vi "AutoAlign_P612_Jan5th2014.vi"() -> ()   [LabVIEW 2014]
uses:
  Controls/StageStates.ctl
panel:
  in  "Align":bool
  in  "Exit":bool
  out "Image":sgl[][](graph)
  out "Aligned":bool
  in  "Repeat":bool
  in  "Quit":bool
  out "Sample":cluster{"X":dbl, "Y":dbl}[](graph)
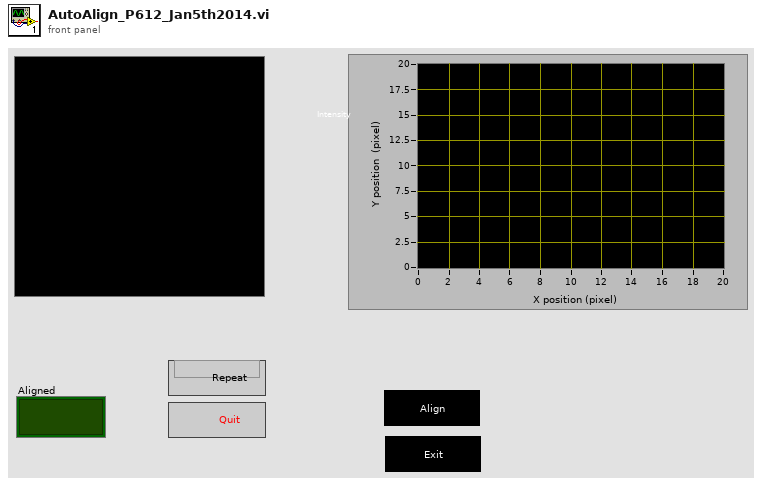
[diagram p1: front panel]
types:
  T1 = typedef "StageStates.ctl" = enum16{"POSITION", "MVR", "MOVE", "HALT", "ONTARGET", "ERROR", "EXIT", "HOME", "ZEROPOS", "NANOPOS", "QUIT", "ANALOG"}
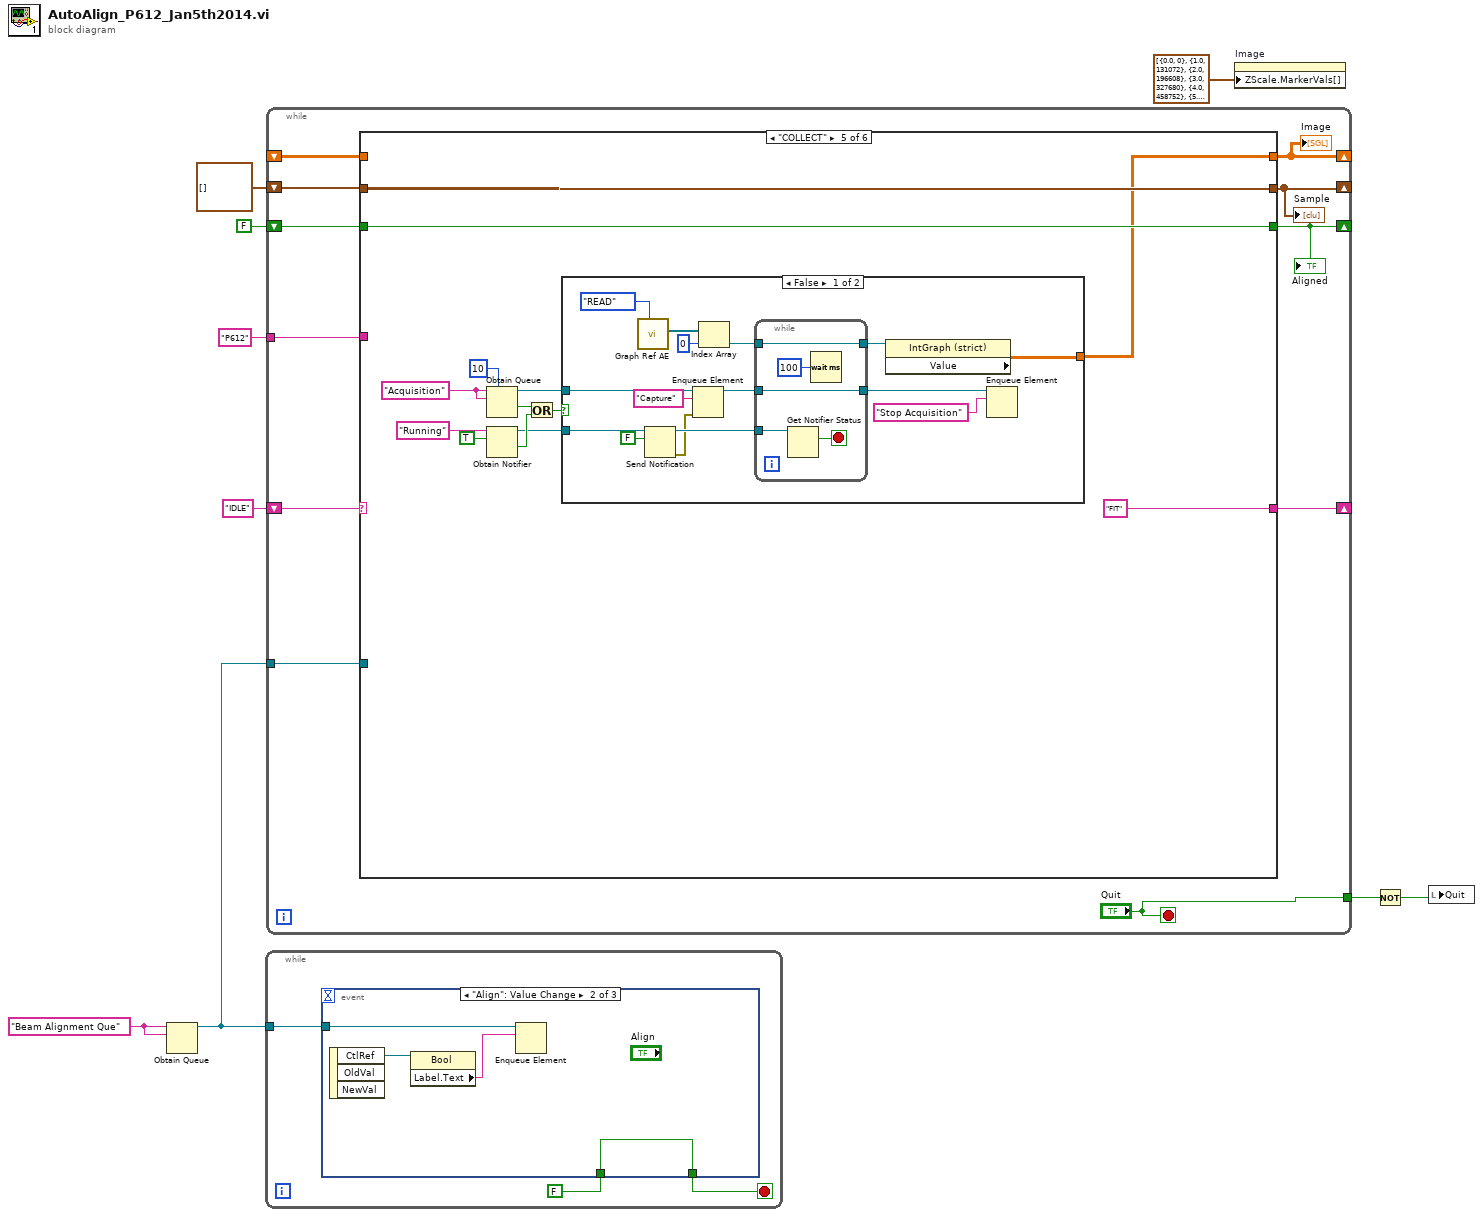
[diagram p0: block diagram]
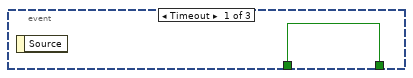
[diagram p2: hidden frame]
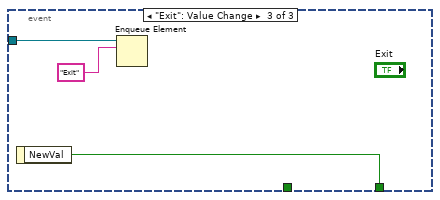
[diagram p3: hidden frame]
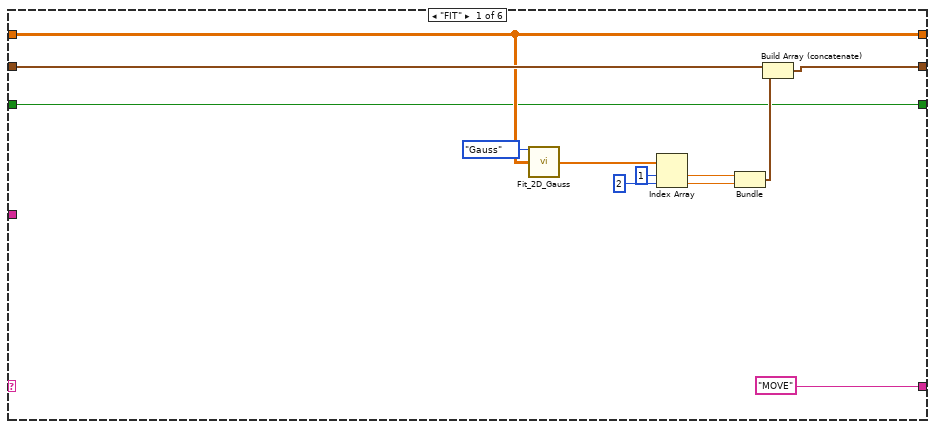
[diagram p4: hidden frame]
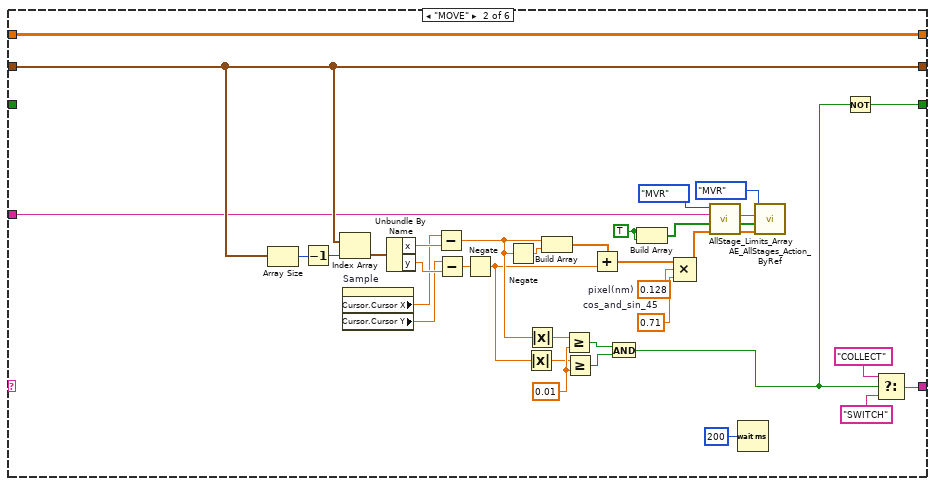
[diagram p5: hidden frame]
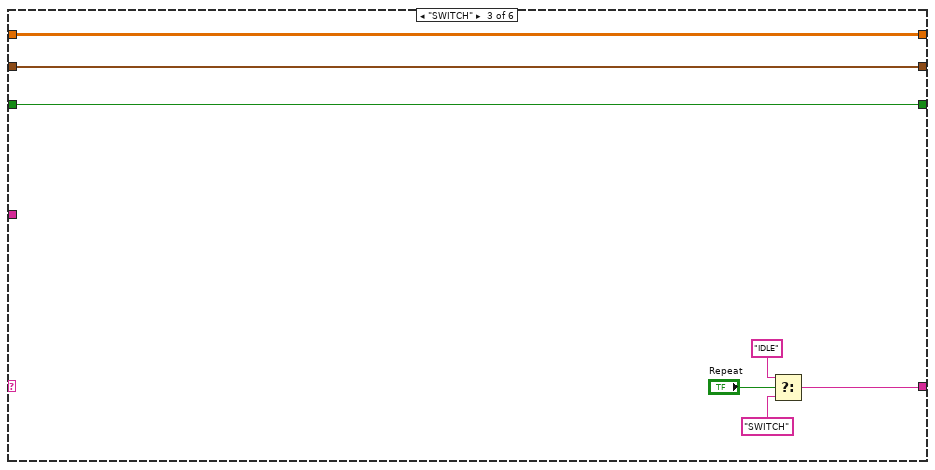
[diagram p6: hidden frame]
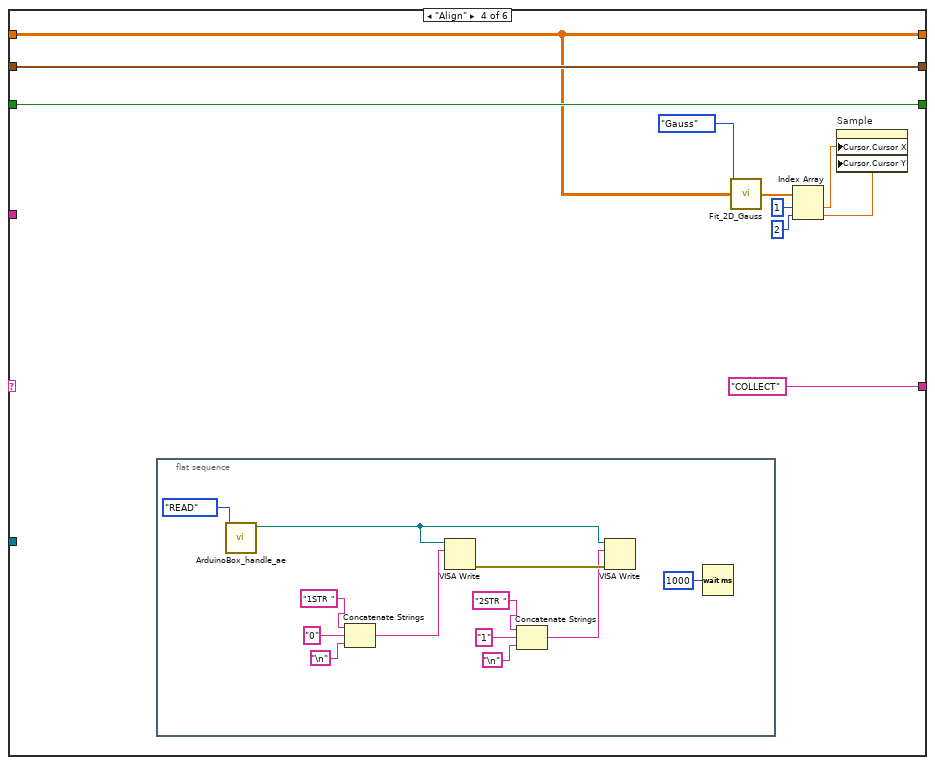
[diagram p7: hidden frame]
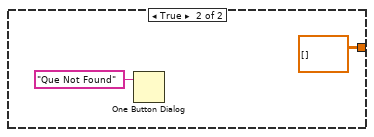
[diagram p8: hidden frame]
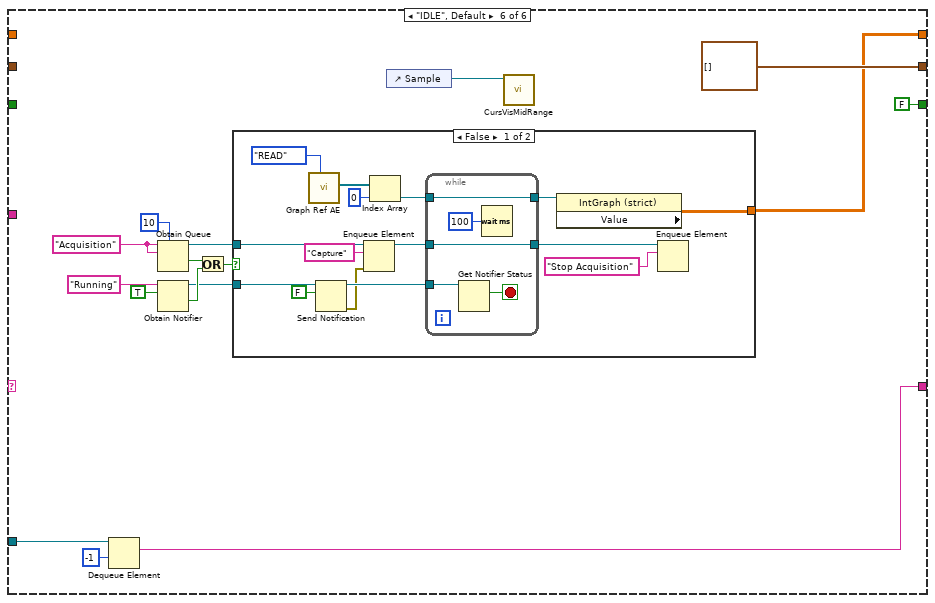
[diagram p9: hidden frame]
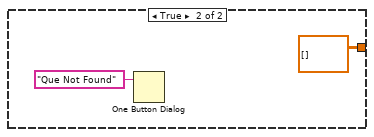
[diagram p10: hidden frame]
diagram:
  w2 = "Beam Alignment Que" ("name (unnamed)")
  n1 = Obtain Queue(name (unnamed)=w2, element data type=w2) -> (queue out=w1:refnum<queue>)  [unwired: 3 in, 2 out]
  n2 = while {
    tunnel: w1 -> [w12]
    stop <- w10 stop-if-true
    n3 = event shown="[1] \"Align\": Value Change" {
      selector: _ -> [_ _ _]
      dyn-events: _ -> [_ _ _]
      timeout: _ -> [_ _ _]
      tunnel: w12 -> [_ w15 w20]
      tunnel: FALSE -> [w13 w14 _]
      tunnel: [w13 w14 w18] -> w10
      event Timeout {
        n4 = event-data() -> ()  [unwired: 1 in, 1 out]
      }
      event "Align": Value Change {
        n5 = event-data() -> ("CtlRef"=w17:refnum<vi>)  [unwired: 1 in, 2 out]
        n6 = property class="Bool"(reference=w17) -> ("Label.Text"=w16:string)  [unwired: 1 in, 2 out]
        n7 = Enqueue Element(queue=w15, element=w16) -> ()  [unwired: 2 in, 3 out]
      }
      event "Exit": Value Change {
        n8 = event-data() -> ("NewVal"=w18:bool)  [unwired: 1 in]
        n9 = Enqueue Element(queue=w20, element="Exit") -> ()  [unwired: 2 in, 3 out]
      }
    }
  }
  n10 = while {
    shift-right: [w22] -> _
    shift-left: _ -> [w31]
    shift-right: [w30] -> _
    shift-left: cluster{"x":dbl, "y":dbl}[] [] ("XY chart data") -> [w24]
    shift-right: [w29] -> _
    shift-left: "IDLE" -> [w26]
    shift-right: [w27] -> _
    shift-left: FALSE -> [w28]
    tunnel: "P612" ("StageID") -> [w25]
    tunnel: ["Quit"] -> w5
    tunnel: w1 -> [w21]
    stop <- "Quit" stop-if-true
    n11 = case shown="\"COLLECT\"" w26 {
      tunnel: [w39 w80 w85 w88 w110 w145] -> w22
      tunnel: w31 -> [w39 w80 w85 w88 _ _]
      tunnel: w24 -> [w41 w54 w86 w95 w122 _]
      tunnel: [w40 w54 w86 w95 w122 cluster{"x":dbl, "y":dbl}[] [] ("XY chart data")] -> w30
      tunnel: w25 -> [_ w47 _ _ _ _]
      tunnel: ["MOVE" w67 w82 "COLLECT" "FIT" w155] -> w29
      tunnel: w28 -> [w37 _ w87 w97 w121 _]
      tunnel: [w37 w52 w87 w97 w121 FALSE] -> w27
      tunnel: w21 -> [_ _ _ _ _ w157]
      frame "FIT" {
        n12 = call "Fit_2D_Gauss.vi"("Enum"=enum16{"Gauss", "Lorentz"}."Gauss", "Image IN"=w39) -> ("Fit Parameters"=w43:dbl[])  [unwired: 12 in, 1 out]
        n13 = Index Array(array=w43, index #1=1 ("index"), index #2=2 ("index")) -> (element #1=w34:dbl, element #2=w33:dbl)
        n14 = Bundle("Numeric"=w34, "Numeric"=w33) -> (w42:cluster{"Numeric":dbl, "Numeric":dbl})  [unwired: 1 in]
        n15 = Build Array (concatenate)(w41, w42) -> (w40:cluster{"Numeric":dbl, "Numeric":dbl}[])
      }
      frame "MOVE" {
        w66 = 0.71  # cos_and_sin_45
        w79 = 0.01 ("y")
        w78 = 0.128  # pixel(nm)
        w77 = TRUE
        n16 = Array Size(array=w54) -> (size(s)=w72:i32)
        n17 = Decrement(x=w72) -> (x-1=w65:i32)
        n18 = Index Array(array=w54, index=w65) -> (element=w73:cluster{"x":dbl, "y":dbl})
        n19 = property on="Sample" class="XYGraph (strict)"() -> ("Cursor.Cursor X"=w71:dbl, "Cursor.Cursor Y"=w70:dbl)  [unwired: 2 in, 2 out]
        n20 = Unbundle By Name(w73) -> ("x"=w74:dbl, "y"=w75:dbl)
        n21 = Subtract(x=w71, y=w74) -> (x-y=w61:dbl)
        n22 = Subtract(x=w70, y=w75) -> (x-y=w62:dbl)
        n23 = Negate(x=w62) -> (-x=w58:dbl)
        n24 = Negate(x=w61) -> (-x=w60:dbl)
        n25 = Absolute Value(x=w58) -> (abs(x)=w63:dbl)
        n26 = Absolute Value(x=w61) -> (abs(x)=w64:dbl)
        n27 = Build Array(w61, w60) -> (w59:dbl[])
        n28 = Greater Or Equal?(x=w64, y=w79) -> (x >= y?=w56:bool)
        n29 = Greater Or Equal?(x=w63, y=w79) -> (x >= y?=w55:bool)
        n30 = Add(x=w59, y=w58) -> (x+y=w57:dbl[])
        n31 = And(x=w56, y=w55) -> (x .and. y?=w53:bool)
        n32 = Build Array(w77, w77) -> (w46:bool[])
        n33 = Compound Arithmetic op=MULTIPLY(w57, w78, w66) -> (w48:dbl[])
        n34 = call "AllStage_Limits_Array.vi"("Step(um)/Position(units)"=w48, "Axis"=w46, "Stage ID"=w47, "MOVE/MVR"=enum16{"MOVE", "MVR"}."MVR") -> ("Positions"=w49:dbl[], "Boolean Array"=w50:bool[], "Stage ID"=w51:string)  [unwired: 5 in]
        n35 = Wait (ms)(milliseconds to wait=u32 200) -> ()  [unwired: 1 out]
        n36 = call "AE_AllStages_Action_ByRef.vi"("Positions"=w49, "Axis"=w50, "Stage ID"=w51, "Action"=StageStates."MVR") -> ()  [unwired: 4 in, 4 out]
        n37 = Not(x=w53) -> (.not. x?=w52:bool)
        n38 = Select(t="COLLECT", s=w53, f="SWITCH") -> (s? t:f=w67:string)
      }
      frame "SWITCH" {
        n39 = Select(t="IDLE", s="Repeat", f="SWITCH") -> (s? t:f=w82:string)
      }
      frame "Align" {
        n40 = flat-sequence {
          frame #0 {
            n41 = call "ArduinoBox_handle_ae.vi"("Enum"=enum16{"WRITE", "READ"}."READ") -> ("VISA resource Out"=w103:refnum<visa-resource-name>)  [unwired: 10 in]
            n42 = Concatenate Strings("1STR ", "0" ("string"), "\n") -> (w106:string)
            n43 = VISA Write(VISA resource name=w103, write buffer=w106) -> (error out=w104:errorcluster)  [unwired: 1 in, 2 out]
            n44 = Concatenate Strings("2STR ", "1" ("string"), "\n") -> (w99:string)
            n45 = VISA Write(VISA resource name=w103, write buffer=w99, error in (no error)=w104) -> ()  [unwired: 3 out]
            n46 = Wait (ms)(milliseconds to wait=u32 1000) -> ()  [unwired: 1 out]
          }
        }
        n47 = call "Fit_2D_Gauss.vi"("Enum"=enum16{"Gauss", "Lorentz"}."Gauss", "Image IN"=w88) -> ("Fit Parameters"=w94:dbl[])  [unwired: 12 in, 1 out]
        n48 = Index Array(array=w94, index #1=1 ("index"), index #2=2 ("index")) -> (element #1=w91:dbl, element #2=w90:dbl)
        n49 = property on="Sample" class="XYGraph (strict)"("Cursor.Cursor X"=w91, "Cursor.Cursor Y"=w90) -> ()  [unwired: 2 in, 2 out]
      }
      frame "COLLECT" {
        w114 = "Acquisition" ("name (unnamed)")
        n50 = Obtain Queue(max queue size (-1, unlimited)=10, name (unnamed)=w114, element data type=w114) -> (queue out=w111:refnum<queue>, created new?=w117:bool)  [unwired: 2 in, 1 out]
        n51 = Obtain Notifier(name (unnamed)="Running", notification data type=TRUE) -> (notifier out=w112:refnum<notifier>, created new?=w118:bool)  [unwired: 2 in, 1 out]
        n52 = Or(x=w117, y=w118) -> (x .or. y?=w119:bool)
        n53 = case shown="False" w119 {
          tunnel: w111 -> [w126 _]
          tunnel: w112 -> [w124 _]
          tunnel: [w123 sgl[][] [] ("Value")] -> w110
          frame False {
            n54 = call "Graph Ref AE.vi"("Action"=enum16{"READ", "WRITE"}."READ") -> ("Graph Ref Out"=w134:refnum<vi>[])  [unwired: 10 in]
            n55 = Send Notification(notification=FALSE, notifier=w124) -> (notifier out=w129:refnum<notifier>, error out=w128:errorcluster)  [unwired: 1 in]
            n56 = Enqueue Element(queue=w126, element="Capture", error in (no error)=w128) -> (queue out=w130:refnum<queue>)  [unwired: 1 in, 2 out]
            n57 = Index Array(array=w134, index=0) -> (element=w136:refnum<vi>)
            n58 = while {
              tunnel: w129 -> [w142]
              tunnel: [w140] -> w131
              tunnel: w130 -> [w140]
              tunnel: [w139] -> w137
              tunnel: w136 -> [w139]
              stop <- w141 stop-if-true
              n59 = Get Notifier Status(notifier=w142) -> (current notification=w141:bool)  [unwired: 1 in, 4 out]
              n60 = Wait (ms)(milliseconds to wait=u32 100) -> ()  [unwired: 1 out]
            }
            n61 = property class="IntGraph (strict)"(reference=w137) -> ("Value"=w123:sgl[][])  [unwired: 1 in, 2 out]
            n62 = Enqueue Element(queue=w131, element="Stop Acquisition" ("f")) -> ()  [unwired: 2 in, 3 out]
          }
          frame True {
            n63 = One Button Dialog(message="Que Not Found") -> ()  [unwired: 1 in, 1 out]
          }
        }
      }
      frame "IDLE", Default {
        w149 = "Acquisition" ("name (unnamed)")
        n64 = Dequeue Element(queue=w157, timeout in ms (-1)=-1) -> (element=w155:string)  [unwired: 1 in, 3 out]
        n65 = Obtain Queue(max queue size (-1, unlimited)=10, name (unnamed)=w149, element data type=w149) -> (queue out=w146:refnum<queue>, created new?=w152:bool)  [unwired: 2 in, 1 out]
        n66 = Obtain Notifier(name (unnamed)="Running", notification data type=TRUE) -> (notifier out=w147:refnum<notifier>, created new?=w153:bool)  [unwired: 2 in, 1 out]
        n67 = Or(x=w152, y=w153) -> (x .or. y?=w154:bool)
        n68 = case shown="False" w154 {
          tunnel: w146 -> [w164 _]
          tunnel: w147 -> [w162 _]
          tunnel: [w161 sgl[][] [] ("Value")] -> w145
          frame False {
            n69 = call "Graph Ref AE.vi"("Action"=enum16{"READ", "WRITE"}."READ") -> ("Graph Ref Out"=w172:refnum<vi>[])  [unwired: 10 in]
            n70 = Send Notification(notification=FALSE, notifier=w162) -> (notifier out=w167:refnum<notifier>, error out=w166:errorcluster)  [unwired: 1 in]
            n71 = Enqueue Element(queue=w164, element="Capture", error in (no error)=w166) -> (queue out=w168:refnum<queue>)  [unwired: 1 in, 2 out]
            n72 = Index Array(array=w172, index=0) -> (element=w174:refnum<vi>)
            n73 = while {
              tunnel: w167 -> [w180]
              tunnel: [w178] -> w169
              tunnel: w168 -> [w178]
              tunnel: [w177] -> w175
              tunnel: w174 -> [w177]
              stop <- w179 stop-if-true
              n74 = Get Notifier Status(notifier=w180) -> (current notification=w179:bool)  [unwired: 1 in, 4 out]
              n75 = Wait (ms)(milliseconds to wait=u32 100) -> ()  [unwired: 1 out]
            }
            n76 = property class="IntGraph (strict)"(reference=w175) -> ("Value"=w161:sgl[][])  [unwired: 1 in, 2 out]
            n77 = Enqueue Element(queue=w169, element="Stop Acquisition" ("f")) -> ()  [unwired: 2 in, 3 out]
          }
          frame True {
            n78 = One Button Dialog(message="Que Not Found") -> ()  [unwired: 1 in, 1 out]
          }
        }
        n79 = control-ref of="Sample"() -> (w159:refnum<vi>)
        n80 = call "CursVisMidRange.vi"("XYGraph in"=w159) -> ()  [unwired: 11 in]
      }
    }
    "Sample" <- w30
    "Aligned" <- w27
    "Image" <- w22
  }
  n81 = property on="Image" class="IntGraph (strict)"("ZScale.MarkerVals[]"=cluster{dbl, u32}[] [{0.0, 0}, {1.0, 131072}, {2.0, 196608}, {3.0, 327680}, {4.0, 458752}, {5.0, 589824}, {6.0, 720896}, {7.0, 851971}, {8.0, 983043}, {9.0, 1114115}, {10.0, 1245187}, {11.0, 1376259}, {12.0, 1507331}, {13.0, 1638403}, {14.0, 1769475}, {15.0, 1769479}, {16.0, 2031623}, {17.0, 2162695}, {18.0, 2293767}, {19.0, 2424839}, {20.0, 2555911}, {21.0, 2686983}, {22.0, 2818055}, {23.0, 2949127}, {24.0, 3080203}, {25.0, 3211275}, {26.0, 3342347}, {27.0, 3473419}, {28.0, 3604491}, {29.0, 3735563}, {30.0, 3866635}, {31.0, 3867403}, {32.0, 4129547}, {33.0, 4260619}, {34.0, 4391691}, {35.0, 4522763}, {36.0, 4653839}, {37.0, 4784911}, {38.0, 4915983}, {39.0, 5178127}, {40.0, 5309199}, {41.0, 5440271}, {42.0, 5571343}, {43.0, 5702415}, {44.0, 5703439}, {45.0, 5965583}, {46.0, 6096655}, {47.0, 6227727}, {48.0, 6358799}, {49.0, 6489871}, {50.0, 6620943}, {51.0, 6752015}, {52.0, 6883087}, {53.0, 7015183}, {54.0, 7146255}, {55.0, 7277327}, {56.0, 7408399}, {57.0, 7539471}, {58.0, 7670543}, {59.0, 7801615}, {60.0, 8063759}, {61.0, 8194831}, {62.0, 8326927}, {63.0, 8457999}, {64.0, 8589075}, {65.0, 8720147}, {66.0, 8851219}, {67.0, 8982291}, {68.0, 9113363}, {69.0, 9114387}, {70.0, 9376531}, {71.0, 9507603}, {72.0, 9638675}, {73.0, 9769747}, {74.0, 9901843}, {75.0, 10032915}, {76.0, 10163987}, {77.0, 10229523}, {78.0, 10295059}, {79.0, 10427155}, {80.0, 10558227}, {81.0, 10689299}, {82.0, 10820371}, {83.0, 10886931}, {84.0, 10952467}, {85.0, 11083539}, {86.0, 11214611}, {87.0, 11215635}, {88.0, 11477779}, {89.0, 11543315}, {90.0, 11608851}, {91.0, 11740947}, {92.0, 11806483}, {93.0, 11872019}, {94.0, 12004115}, {95.0, 12135187}, {96.0, 12266259}, {97.0, 12267283}, {98.0, 12398355}, {99.0, 12529427}, {100.0, 12530451}, {101.0, 12595987}, {102.0, 12530451}, {103.0, 12793619}, {104.0, 12794131}, {105.0, 12794643}, {106.0, 13056787}, {107.0, 13057299}, {108.0, 13057811}, {109.0, 13188883}, {110.0, 13320979}, {111.0, 13386515}, {112.0, 13452563}, {113.0, 13584147}, {114.0, 13584659}, {115.0, 13585171}, {116.0, 13585683}, {117.0, 13717267}, {118.0, 13848339}, {119.0, 13849363}, {120.0, 13849875}, {121.0, 13850387}, {122.0, 13981459}, {123.0, 14113555}, {124.0, 14114067}, {125.0, 14114579}, {126.0, 14115091}, {127.0, 14246675}, {128.0, 14377747}, {129.0, 14378771}, {130.0, 14379283}, {131.0, 14379539}, {132.0, 14379795}, {133.0, 14380819}, {134.0, 14511891}, {135.0, 14643987}, {136.0, 14644503}, {137.0, 14645015}, {138.0, 14645527}, {139.0, 14646039}, {140.0, 14646551}, {141.0, 14778135}, {142.0, 14909207}, {143.0, 14910231}, {144.0, 14910747}, {145.0, 14911259}, {146.0, 14911771}, {147.0, 14912283}, {148.0, 14912797}, {149.0, 15044383}, {150.0, 15175455}, {151.0, 15175967}, {152.0, 15176479}, {153.0, 15176991}, {154.0, 15177507}, {155.0, 15178019}, {156.0, 15178531}, {157.0, 15310115}, {158.0, 15441701}, {159.0, 15441959}, {160.0, 15442215}, {161.0, 15442727}, {162.0, 15443243}, {163.0, 15443755}, {164.0, 15444269}, {165.0, 15444783}, {166.0, 15444783}, {167.0, 15576367}, {168.0, 15707953}, {169.0, 15708467}, {170.0, 15708979}, {171.0, 15708981}, {172.0, 15708983}, {173.0, 15710011}, {174.0, 15710523}, {175.0, 15711037}, {176.0, 15711039}, {177.0, 15711553}, {178.0, 15843139}, {179.0, 15974213}, {180.0, 15974215}, {181.0, 15974217}, {182.0, 15974219}, {183.0, 15975755}, {184.0, 15976271}, {185.0, 15976785}, {186.0, 15977299}, {187.0, 15977301}, {188.0, 15977815}, {189.0, 15978327}, {190.0, 15978331}, {191.0, 16109917}, {192.0, 16241503}, {193.0, 16241505}, {194.0, 16242019}, {195.0, 16242535}, {196.0, 16242537}, {197.0, 16242539}, {198.0, 16243563}, {199.0, 16243567}, {200.0, 16244081}, {201.0, 16244595}, {202.0, 16244599}, {203.0, 16244601}, {204.0, 16244603}, {205.0, 16245627}, {206.0, 16245631}, {207.0, 16245633}, {208.0, 16246147}, {209.0, 16246663}, {210.0, 16377735}, {211.0, 16508811}, {212.0, 16508815}, {213.0, 16509839}, {214.0, 16509843}, {215.0, 16509845}, {216.0, 16509847}, {217.0, 16510361}, {218.0, 16510875}, {219.0, 16510879}, {220.0, 16510881}, {221.0, 16510883}, {222.0, 16511399}, {223.0, 16511911}, {224.0, 16511915}, {225.0, 16511917}, {226.0, 16511919}, {227.0, 16511923}, {228.0, 16512437}, {229.0, 16512951}, {230.0, 16512955}, {231.0, 16512957}, {232.0, 16512959}, {233.0, 16512961}, {234.0, 16512963}, {235.0, 16512967}, {236.0, 16513481}, {237.0, 16513995}, {238.0, 16513999}, {239.0, 16514001}, {240.0, 16514003}, {241.0, 16514005}, {242.0, 16514007}, {243.0, 16514011}, {244.0, 16514013}, {245.0, 16514015}, {246.0, 16514019}, {247.0, 16514021}, {248.0, 16514023}, {249.0, 16514027}, {250.0, 16514029}, {251.0, 16514031}, {252.0, 16514035}, {253.0, 16514037}, {254.0, 16514039}, {255.0, 16514043}] ("Z Scale.Marker Values[]")) -> ()  [unwired: 2 in, 2 out]
  n82 = Not(x=w5) -> (.not. x?=w4:bool)
  n83 = local write "Quit"(w4) -> ()
